vi "Pattern Reorder.vi"(10 "write data (0x0000) in":u32, 11 "channel list (all:\"\")":string) -> (2 "write mask":u32, 3 "write data final":u32)   [LabVIEW 2019]
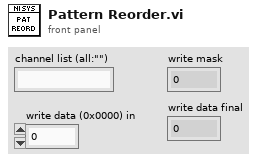
[diagram p1: front panel]
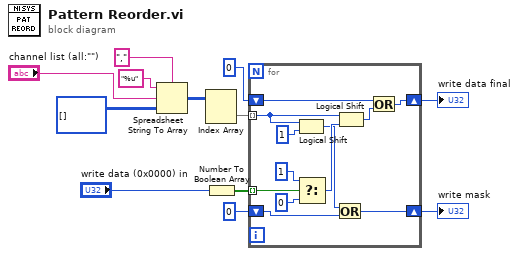
[diagram p0: block diagram]
diagram:
  n1 = Spreadsheet String To Array(delimiter (Tab)=",", format string="%u" ("delimiter (Tab)"), spreadsheet string="channel list (all:\"\")", array type (2D Dbl)=u32[][] []) -> (array=w5:u32[][])
  n2 = Index Array(array=w5) -> (element=w7:u32[])  [unwired: 2 in]
  n3 = Number To Boolean Array(number="write data (0x0000) in") -> (Boolean array=w4:bool[])
  n4 = for {
    tunnel: w4 -> [w21] mode=indexing
    shift-right: [w23] -> w9
    shift-left: u32 0 ("write data (0x0000)") -> [w24]
    tunnel: w7 -> [w17] mode=indexing
    shift-right: [w13] -> w1
    shift-left: u32 0 ("write data (0x0000)") -> [w14]
    n5 = Logical Shift(y=w17, x=u32 1) -> (x << y=w15:u32)
    n6 = Select(t=u32 1, s=w21, f=u32 0) -> (s? t:f=w19:u32)
    n7 = Or(x=w15, y=w14) -> (x .or. y?=w13:u32)
    n8 = Logical Shift(y=w17, x=w19) -> (x << y=w22:u32)
    n9 = Or(x=w24, y=w22) -> (x .or. y?=w23:u32)
  }
  "write data final" <- w9
  "write mask" <- w1
